vi "TPI set power.vi"(8 "Error in (no error)":errorcluster, 9 "power (dBm)":i32=-10, 11 "VISA resource name":refnum<visa-resource-name>) -> (0 "Error out":errorcluster, 3 "VISA resource name out":refnum<visa-resource-name>)   [LabVIEW 2020]
panel:
  # "coerce power to be between -90 dBm and 10 dBm"
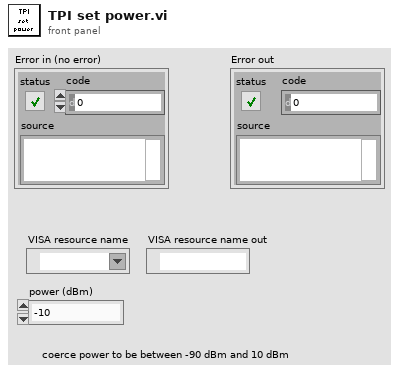
[diagram p1: front panel]
types:
  T1 = enum16{"big-endian, network order", "native, host order", "little-endian"}
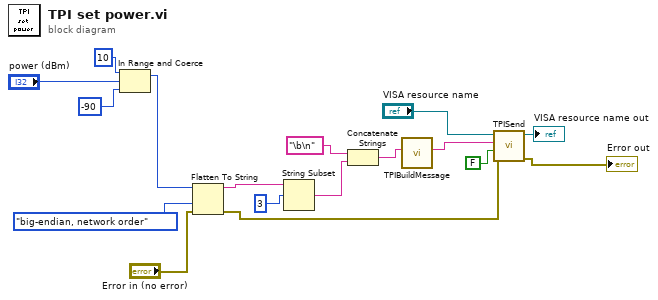
[diagram p0: block diagram]
diagram:
  n1 = In Range and Coerce(upper limit=10, x="power (dBm)", lower limit=-90 ("upper limit")) -> (coerced(x)=w7:i32)  [unwired: 1 out]
  n2 = Flatten To String(anything=w7, byte order (0:big-endian, network order)=T1."big-endian, network order", error in (no error)="Error in (no error)") -> (data string=w16:string, error out=w2:errorcluster)  [unwired: 1 in, 1 out]
  n3 = String Subset(string=w16, offset (0)=3) -> (substring=w13:string)  [unwired: 1 in]
  n4 = Concatenate Strings("\b\n" ("Command"), w13) -> (w10:string)
  n5 = call "TPIBuildMessage.vi"("Command"=w10) -> ("Message"=w11:string)  [unwired: 10 in]
  n6 = call "TPISend.vi"("error in (no error)"=w2, "Read Responce"=FALSE, "write buffer"=w11, "VISA resource name"="VISA resource name") -> ("error out"=→"Error out":errorcluster, "VISA resource name out"=→"VISA resource name out":refnum<visa-resource-name>)  [unwired: 5 in, 1 out]
